vi "CRYShow Name Changing Dialog.vi"(11 "Detail Information In":string[][](array[string])) -> ()   [LabVIEW 2013]
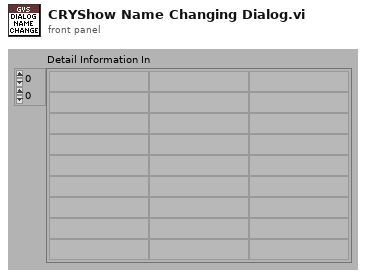
[diagram p1: front panel]
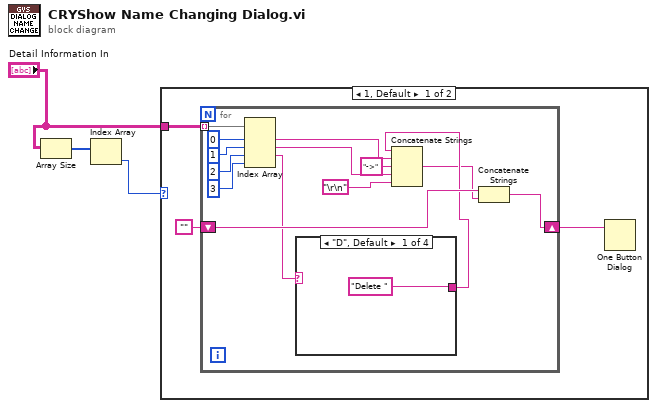
[diagram p0: block diagram]
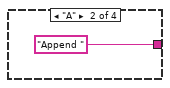
[diagram p2: hidden frame]
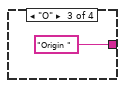
[diagram p3: hidden frame]
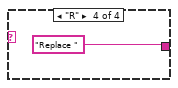
[diagram p4: hidden frame]
diagram:
  n1 = Array Size(array="Detail Information In") -> (size(s)=w3:i32[])
  n2 = Index Array(array=w3) -> (element=w2:i32)  [unwired: 1 in]
  n3 = case shown="1, Default" w2 {
    tunnel: "Detail Information In" -> [w5 _]
    frame 1, Default {
      n4 = for {
        shift-right: [w7] -> w4
        shift-left: "" -> [w20]
        tunnel: w5 -> [w19] mode=indexing
        n5 = Index Array(array=w19, index #1=0 ("index"), index #2=1 ("index"), index #3=2 ("index"), index #4=3 ("index")) -> (element #1=w14:string, element #2=w13:string, element #3=w11:string)  [unwired: 1 out]
        n6 = case shown="\"D\", Default" w11 {
          tunnel: ["Delete " "Append " ("string") "Origin " ("string") "Replace " ("string")] -> w10
          frame "D", Default {
          }
          frame "A" {
          }
          frame "O" {
          }
          frame "R" {
          }
        }
        n7 = Concatenate Strings(w10, w14, "->" ("string"), w13, "\r\n") -> (w8:string)
        n8 = Concatenate Strings(w20, w8) -> (w7:string)
      }
      n9 = One Button Dialog(message=w4) -> ()  [unwired: 1 in, 1 out]
    }
    frame 0 {
    }
  }
